vi "Part 1.vi"(11 "Input":string) -> (3 "Output":i64)   [LabVIEW 2021]
uses:
  0e1cb530-612f-43b5-ac3a-243a7e2c5b19.vi
  <userlib>/_OpenG.lib/string/string.llb/Convert EOLs (String)__ogtk.vi
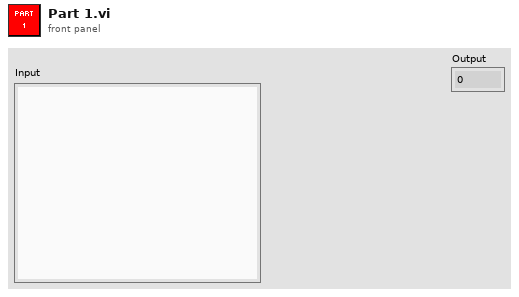
[diagram p1: front panel]
types:
  T1 = set{cluster{"row":i32, "col":i32, "dir":enum16{"right", "left", "up", "down"}}}
  T2 = cluster{"row":i32, "col":i32, "dir":enum16{"right", "left", "up", "down"}}
  T3 = cluster{"row":i32, "col":i32, "dir":enum16{"right", "left", "up", "down"}}[]
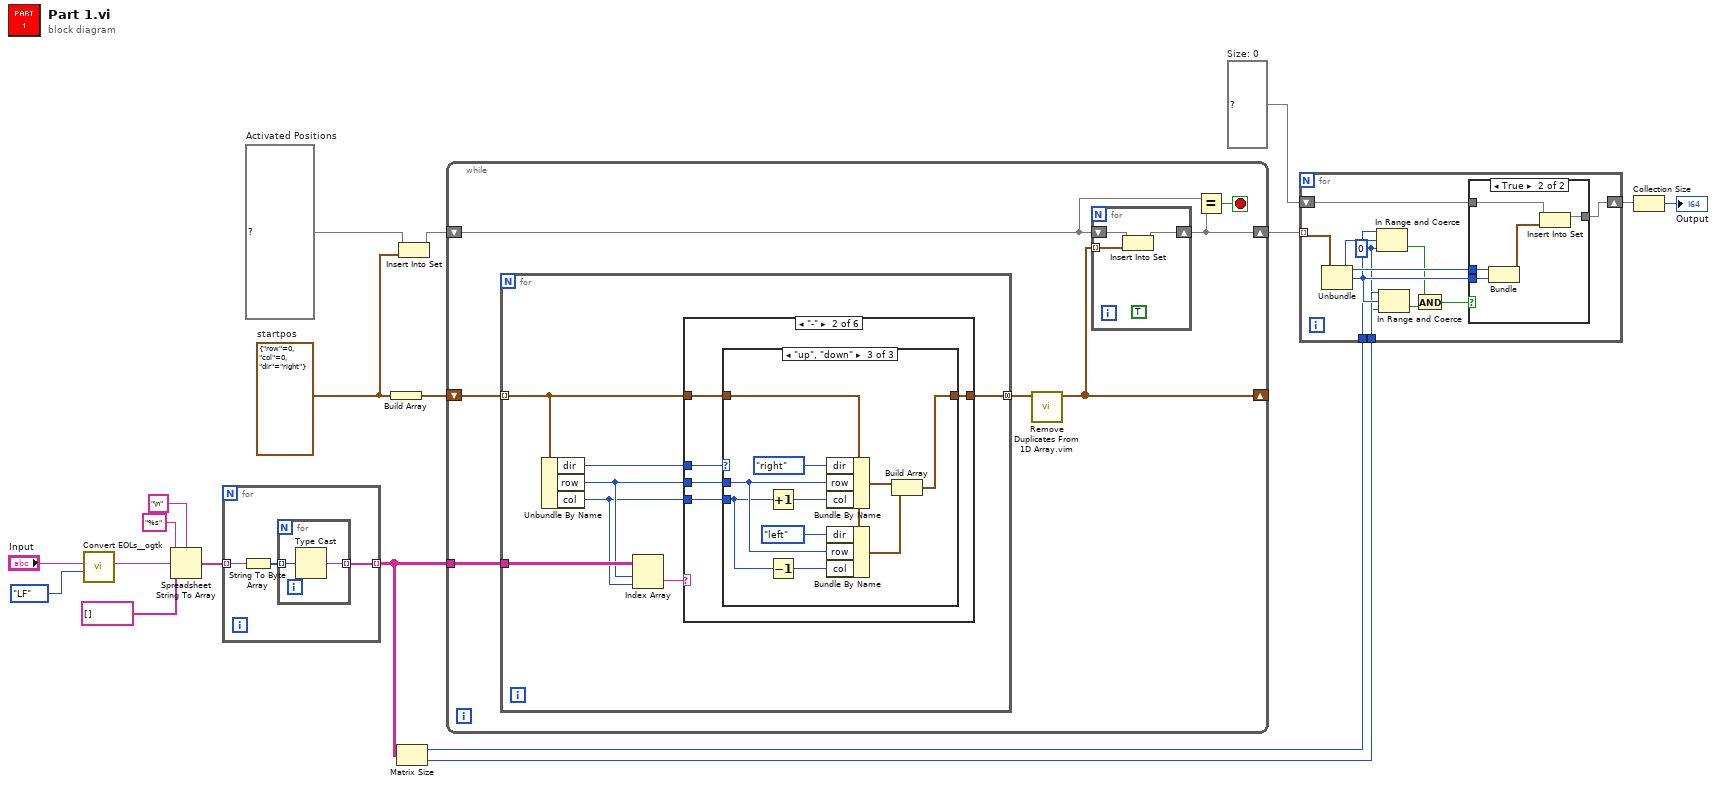
[diagram p0: block diagram]
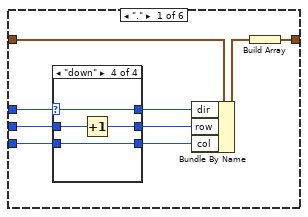
[diagram p2: hidden frame]
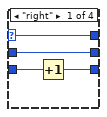
[diagram p3: hidden frame]
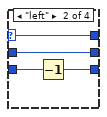
[diagram p4: hidden frame]
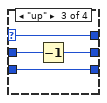
[diagram p5: hidden frame]
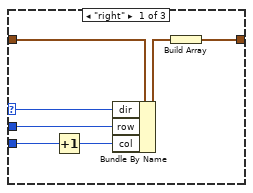
[diagram p6: hidden frame]
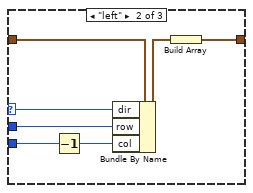
[diagram p7: hidden frame]
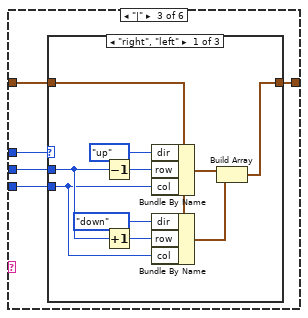
[diagram p8: hidden frame]
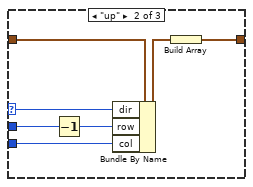
[diagram p9: hidden frame]
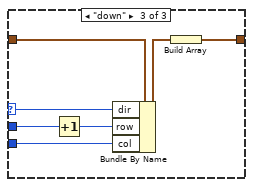
[diagram p10: hidden frame]
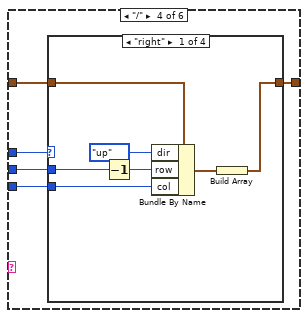
[diagram p11: hidden frame]
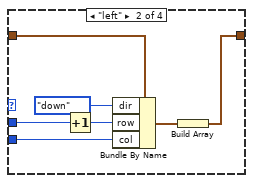
[diagram p12: hidden frame]
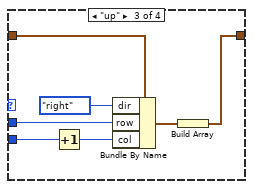
[diagram p13: hidden frame]
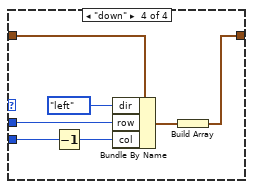
[diagram p14: hidden frame]
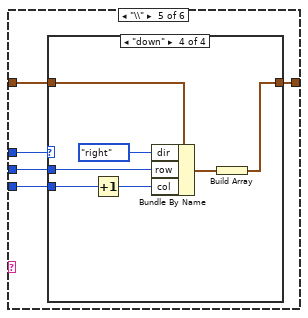
[diagram p15: hidden frame]
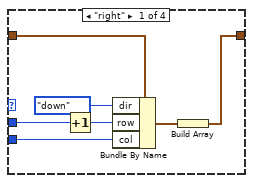
[diagram p16: hidden frame]
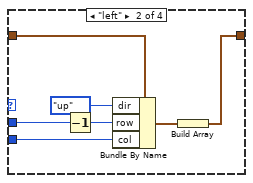
[diagram p17: hidden frame]
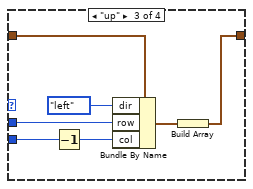
[diagram p18: hidden frame]
diagram:
  w2 = set{cluster{"row":i32, "col":i32}} {}  # Size: 0
  w10 = T1 {}  # Activated Positions
  w8 = T2 {"row"=0, "col"=0, "dir"=enum."right"}  # startpos
  n1 = call-poly <userlib>:"Convert EOLs__ogtk.vi"("Convert to:"=enum16{"CR", "LF", "CRLF"}."LF", "String in"="Input") -> ("String out"=w14:string)  [unwired: 9 in]
  n2 = Spreadsheet String To Array(delimiter (Tab)="\n", format string="%s", spreadsheet string=w14, array type (2D Dbl)=string[] []) -> (array=w12:string[])
  n3 = for {
    tunnel: w12 -> [w21] mode=indexing
    tunnel: [w19] -> w7 mode=indexing
    n4 = String To Byte Array(string=w21) -> (unsigned byte array=w20:u8[])
    n5 = for {
      tunnel: w20 -> [w23] mode=indexing
      tunnel: [w22] -> w19 mode=indexing
      n6 = Type Cast(x=w23) -> (*(type *) &x=w22:string)  [unwired: 1 in]
    }
  }
  n7 = Build Array(w8) -> (w11:T3)
  n8 = Matrix Size(0:w7) -> (1:w4:i32, 2:w1:i32)
  n9 = Insert Into Set(10:w8, 11:w10) -> (3:w9:T1)  [unwired: 1 out]
  n10 = while {
    shift-right: [w29] -> w6
    shift-left: w9 -> [w28]
    shift-right: [w24] -> _
    shift-left: w11 -> [w27]
    tunnel: w7 -> [w25]
    stop <- w30 stop-if-true
    n11 = for {
      tunnel: w27 -> [w34] mode=indexing
      tunnel: [w35] -> w26 mode=concatenating
      tunnel: w25 -> [w37]
      n12 = Unbundle By Name(w34) -> ("dir"=w33:enum16{"right", "left", "up", "down"}, "row"=w32:i32, "col"=w31:i32)
      n13 = Index Array(array=w37, index (row)=w32, index (col)=w31) -> (element=w36:string)
      n14 = case shown="\"-\"" w36 {
        tunnel: w32 -> [w42 w65 w94 w123 w156 _]
        tunnel: w31 -> [w40 w64 w93 w122 w155 _]
        tunnel: w33 -> [w43 w66 w95 w124 w157 _]
        tunnel: w34 -> [w46 w67 w96 w125 w158 _]
        tunnel: [w45 w63 w92 w121 w154 _] -> w35
        frame "." {
          n15 = case shown="\"down\"" w43 {
            selector: w43 -> [w47 w51 w55 w59]
            tunnel: w42 -> [w50 w54 w57 w61]
            tunnel: w40 -> [w49 w53 w58 w62]
            tunnel: [w50 w54 w56 w60] -> w39
            tunnel: [w48 w52 w58 w62] -> w41
            tunnel: [w47 w51 w55 w59] -> w38
            frame "right" {
              n16 = Increment(x=w49) -> (x+1=w48:i32)
            }
            frame "left" {
              n17 = Decrement(x=w53) -> (x-1=w52:i32)
            }
            frame "up" {
              n18 = Decrement(x=w57) -> (x-1=w56:i32)
            }
            frame "down" {
              n19 = Increment(x=w61) -> (x+1=w60:i32)
            }
          }
          n20 = Bundle By Name(cluster=w46, "dir"=w38, "row"=w39, "col"=w41) -> (w44:T2)
          n21 = Build Array(w44) -> (w45:T3)
        }
        frame "-" {
          n22 = case shown="\"up\", \"down\"" w66 {
            selector: w66 -> [w73 w80 _]
            tunnel: w67 -> [w74 w81 w83]
            tunnel: w65 -> [w72 w79 w85]
            tunnel: w64 -> [w71 w78 w84]
            tunnel: [w69 w76 w91] -> w63
            frame "right" {
              n23 = Increment(x=w71) -> (x+1=w68:i32)
              n24 = Bundle By Name(cluster=w74, "dir"=w73, "row"=w72, "col"=w68) -> (w70:T2)
              n25 = Build Array(w70) -> (w69:T3)
            }
            frame "left" {
              n26 = Decrement(x=w78) -> (x-1=w75:i32)
              n27 = Bundle By Name(cluster=w81, "dir"=w80, "row"=w79, "col"=w75) -> (w77:T2)
              n28 = Build Array(w77) -> (w76:T3)
            }
            frame "up", "down" {
              n29 = Increment(x=w84) -> (x+1=w89:i32)
              n30 = Decrement(x=w84) -> (x-1=w88:i32)
              n31 = Bundle By Name(cluster=w83, "dir"=enum16{"right", "left", "up", "down"}."right", "row"=w85, "col"=w89) -> (w86:T2)
              n32 = Bundle By Name(cluster=w83, "dir"=enum16{"right", "left", "up", "down"}."left", "row"=w85, "col"=w88) -> (w82:T2)
              n33 = Build Array(w86, w82) -> (w91:T3)
            }
          }
        }
        frame "|" {
          n34 = case shown="\"right\", \"left\"" w95 {
            selector: w95 -> [_ w112 w119]
            tunnel: w96 -> [w100 w113 w120]
            tunnel: w94 -> [w102 w111 w118]
            tunnel: w93 -> [w101 w110 w117]
            tunnel: [w106 w108 w115] -> w92
            frame "right", "left" {
              n35 = Decrement(x=w102) -> (x-1=w98:i32)
              n36 = Increment(x=w102) -> (x+1=w97:i32)
              n37 = Bundle By Name(cluster=w100, "dir"=enum16{"right", "left", "up", "down"}."up", "row"=w98, "col"=w101) -> (w103:T2)
              n38 = Bundle By Name(cluster=w100, "dir"=enum16{"right", "left", "up", "down"}."down", "row"=w97, "col"=w101) -> (w99:T2)
              n39 = Build Array(w103, w99) -> (w106:T3)
            }
            frame "up" {
              n40 = Decrement(x=w111) -> (x-1=w107:i32)
              n41 = Bundle By Name(cluster=w113, "dir"=w112, "row"=w107, "col"=w110) -> (w109:T2)
              n42 = Build Array(w109) -> (w108:T3)
            }
            frame "down" {
              n43 = Increment(x=w118) -> (x+1=w114:i32)
              n44 = Bundle By Name(cluster=w120, "dir"=w119, "row"=w114, "col"=w117) -> (w116:T2)
              n45 = Build Array(w116) -> (w115:T3)
            }
          }
        }
        frame "/" {
          n46 = case shown="\"right\"" w124 {
            tunnel: w125 -> [w127 w134 w141 w148]
            tunnel: w123 -> [w129 w136 w143 w150]
            tunnel: w122 -> [w128 w135 w142 w149]
            tunnel: [w132 w139 w146 w153] -> w121
            frame "right" {
              n47 = Decrement(x=w129) -> (x-1=w126:i32)
              n48 = Bundle By Name(cluster=w127, "dir"=enum16{"right", "left", "up", "down"}."up", "row"=w126, "col"=w128) -> (w130:T2)
              n49 = Build Array(w130) -> (w132:T3)
            }
            frame "left" {
              n50 = Increment(x=w136) -> (x+1=w133:i32)
              n51 = Bundle By Name(cluster=w134, "dir"=enum16{"right", "left", "up", "down"}."down", "row"=w133, "col"=w135) -> (w137:T2)
              n52 = Build Array(w137) -> (w139:T3)
            }
            frame "up" {
              n53 = Increment(x=w142) -> (x+1=w140:i32)
              n54 = Bundle By Name(cluster=w141, "dir"=enum16{"right", "left", "up", "down"}."right", "row"=w143, "col"=w140) -> (w144:T2)
              n55 = Build Array(w144) -> (w146:T3)
            }
            frame "down" {
              n56 = Decrement(x=w149) -> (x-1=w147:i32)
              n57 = Bundle By Name(cluster=w148, "dir"=enum16{"right", "left", "up", "down"}."left", "row"=w150, "col"=w147) -> (w151:T2)
              n58 = Build Array(w151) -> (w153:T3)
            }
          }
        }
        frame "\\" {
          n59 = case shown="\"down\"" w157 {
            tunnel: w158 -> [w160 w167 w174 w181]
            tunnel: w156 -> [w162 w169 w176 w183]
            tunnel: w155 -> [w161 w168 w175 w182]
            tunnel: [w165 w172 w179 w186] -> w154
            frame "right" {
              n60 = Increment(x=w162) -> (x+1=w159:i32)
              n61 = Bundle By Name(cluster=w160, "dir"=enum16{"right", "left", "up", "down"}."down", "row"=w159, "col"=w161) -> (w163:T2)
              n62 = Build Array(w163) -> (w165:T3)
            }
            frame "left" {
              n63 = Decrement(x=w169) -> (x-1=w166:i32)
              n64 = Bundle By Name(cluster=w167, "dir"=enum16{"right", "left", "up", "down"}."up", "row"=w166, "col"=w168) -> (w170:T2)
              n65 = Build Array(w170) -> (w172:T3)
            }
            frame "up" {
              n66 = Decrement(x=w175) -> (x-1=w173:i32)
              n67 = Bundle By Name(cluster=w174, "dir"=enum16{"right", "left", "up", "down"}."left", "row"=w176, "col"=w173) -> (w177:T2)
              n68 = Build Array(w177) -> (w179:T3)
            }
            frame "down" {
              n69 = Increment(x=w182) -> (x+1=w180:i32)
              n70 = Bundle By Name(cluster=w181, "dir"=enum16{"right", "left", "up", "down"}."right", "row"=w183, "col"=w180) -> (w184:T2)
              n71 = Build Array(w184) -> (w186:T3)
            }
          }
        }
        frame "", Default {
        }
      }
    }
    n72 = call "Remove Duplicates From 1D Array.vim"("array"=w26) -> ("array with duplicates removed"=w24:T3)  [unwired: 10 in]
    n73 = for {
      shift-right: [w188] -> w29
      shift-left: w28 -> [w189]
      tunnel: w24 -> [w187] mode=indexing
      (unwired) TRUE
      n74 = Insert Into Set(10:w187, 11:w189) -> (3:w188:T1)  [unwired: 1 out]
    }
    n75 = Equal?(x=w28, y=w29) -> (x = y?=w30:bool)
  }
  n76 = for {
    tunnel: w6 -> [w200] mode=indexing
    shift-right: [w199] -> w5
    shift-left: w2 -> [w198]
    tunnel: w4 -> [w192]
    tunnel: w1 -> [w191]
    w190 = 0 ("lower limit")
    n77 = Unbundle(w200) -> ("row"=w197:i32, "col"=w196:i32)  [unwired: 1 out]
    n78 = In Range and Coerce(upper limit=w192, x=w197, lower limit=w190) -> (In Range?=w194:bool)  [unwired: 1 out]
    n79 = In Range and Coerce(upper limit=w191, x=w196, lower limit=w190) -> (In Range?=w195:bool)  [unwired: 1 out]
    n80 = And(x=w194, y=w195) -> (x .and. y?=w193:bool)
    n81 = case shown="True" w193 {
      tunnel: w197 -> [_ w206]
      tunnel: w196 -> [_ w205]
      tunnel: [w201 w203] -> w199
      tunnel: w198 -> [w201 w202]
      frame False {
      }
      frame True {
        n82 = Bundle("row"=w206, "col"=w205) -> (w204:cluster{"row":i32, "col":i32})  [unwired: 1 in]
        n83 = Insert Into Set(10:w204, 11:w202) -> (3:w203:set{cluster{"row":i32, "col":i32}})  [unwired: 1 out]
      }
    }
  }
  n84 = Collection Size(1:w5) -> (0:→"Output":i32)
